vi "Subvi_JoystickRamping_Teleop.vi"(8 "error in (no error)":errorcluster, 10 "threshold":dbl=0.1 format="%#_13g", 11 "VoltageIn":dbl) -> (0 "error out":errorcluster, 3 "voltage out":dbl)   [LabVIEW 2017]
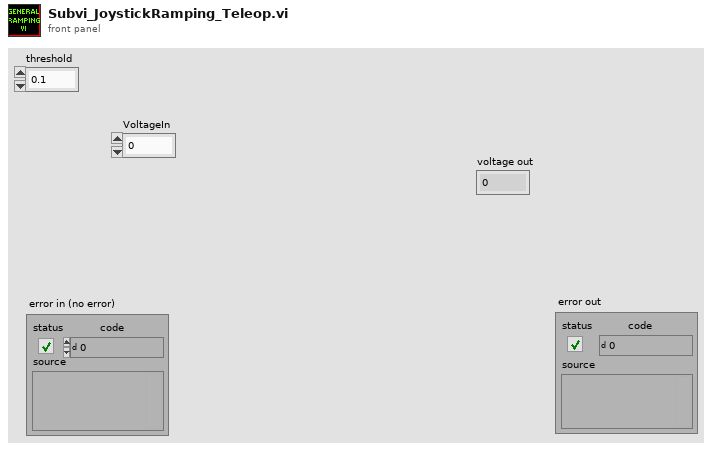
[diagram p1: front panel]
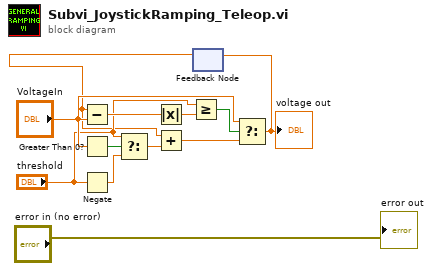
[diagram p0: block diagram]
diagram:
  n1 = Greater Than 0?(x="VoltageIn") -> (x > 0?=w7:bool)
  n2 = Negate(x="threshold") -> (-x=w5:dbl)
  n3 = Select(t="threshold", s=w7, f=w5) -> (s? t:f=w4:dbl)
  n4 = feedback #1() -> (w2:dbl)  [unwired: 1 in]
  n5 = Subtract(x=w2, y="VoltageIn") -> (x-y=w11:dbl)
  n6 = Absolute Value(x=w11) -> (abs(x)=w10:dbl)
  n7 = Add(x=w2, y=w4) -> (x+y=w3:dbl)
  n8 = Greater Or Equal?(x="threshold", y=w10) -> (x >= y?=w9:bool)
  n9 = Select(t="VoltageIn", s=w9, f=w3) -> (s? t:f=w12:dbl)
  "voltage out" <- w12
  n10 = feedback-in #1(w12) -> ()
  "error out" <- "error in (no error)"
